vi "Get SNAME.vi"(8 "error in":errorcluster, 10 "Element Branch In":refnum<class "Tree.lvclass">, 11 "Referential in":refnum<class "Referential.lvclass">) -> (0 "error out":errorcluster, 2 "Element Branch Out":refnum<class "Tree.lvclass">, 3 "Referential out":refnum<class "Referential.lvclass">)   [LabVIEW 2019, in "ParseGDSII.lvclass"]
uses:
  ParseGDSII.lvclass
  Elements/Referential.lvclass
  Tree/Tree.lvclass
  DataTypes/Base/GDSII.DataType.lvclass
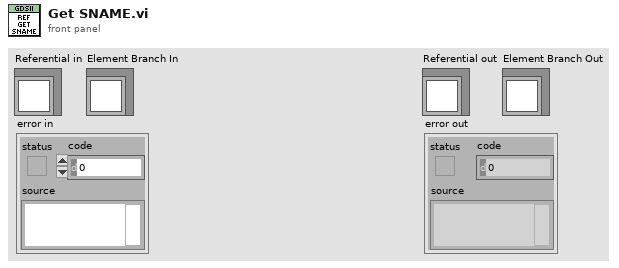
[diagram p1: front panel]
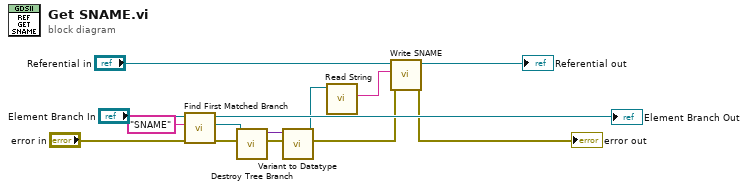
[diagram p0: block diagram]
diagram:
  n1 = call "Find First Matched Branch.vi"("error in"="error in", "Branch Name Exact"="SNAME", "Tree in"="Element Branch In") -> ("error out"=w14:errorcluster, "Matched Branch"=w12:refnum<class "Tree.lvclass">, "Tree out"=→"Element Branch Out":refnum<class "Tree.lvclass">)  [unwired: 5 in, 1 out]
  n2 = call "Destroy Tree Branch.vi"("error in"=w14, "Tree in"=w12) -> ("error out"=w13:errorcluster, "Root"=w11:variant)  [unwired: 8 in]
  n3 = call "Variant to Datatype.vi"("error in"=w13, "Variant"=w11) -> ("error out"=w8:errorcluster, "DataType"=w7:refnum<class "GDSII.DataType.lvclass">)  [unwired: 8 in]
  n4 = call-dynamic "Read String.vi"("GDSII.DataType in"=w7) -> ("String"=w6:string)  [unwired: 9 in, 1 out]
  n5 = call-dynamic "Write SNAME.vi"("error in (no error)"=w8, "SNAME"=w6, "Referential in"="Referential in") -> ("error out"=→"error out":errorcluster, "Referential out"=→"Referential out":refnum<class "Referential.lvclass">)  [unwired: 7 in]
